vi "Format HF Cell.vi"(0 "PdfP Cell":refnum<k24>, 2 "Header or Footer":T1=enum."Footer", 5 "Header Footer Cluster with references":T2={"Start page"=1, "Type"=enum."Select", "Start with #"=1, "Alignment"=enum."Center", "Vertical Alignement"=enum."MIDDLE", "Page #"={"Text 1"="", "Text 2"="", "Text 3"=""}, "Text"=refnum, "Scaled Img"=refnum, "PdfPCell"=refnum, "PdfPTable"=refnum, "Font Cluster"={"Name"="", "Size"=-1.0, "Color"=0, "Style"={"Bold"=FALSE, "Italic"=FALSE, "Underline"=FALSE, "Strikeout"=FALSE}, "Type"={"Type&direction"=enum."Select", "Embedded"=FALSE, "Encoding"=""}}, "Font "=refnum, "Img (%)"=100.0, "Line"={"Line"=enum."Horizontal line", "Thickness (points)"=0.75, "Colour"=7171459}, "Line spacing"=enum."Select"}, 7 "Padding (points)":sgl, 9 "FixedHeight (points)":sgl, 11 "error in (no error)":errorcluster) -> (4 "PdfP Cell duplicate":refnum<k24>, 15 "error out":errorcluster)   [LabVIEW 2019]
doc: "Version 2.0\nDeveloped by Jean-Marc Simard\nCopyright © 2012, Exaprom Inc.\nAll rights reserved.\nLicense: BSD\n\nWith iTextSharp 4.1.6 (http://itextsharp.sourceforge.net)\nunder Mozilla Public License Version 1.1\n(http://www.mozilla.org/MPL/MPL-1.1.html)"
uses:
  C:/Program Files/National Instruments/LabVIEW 2019/user.lib/Exaprom PDF/DLL/itextsharp.dll
  DLL/itextsharp.dll
  <userlib>/Exaprom PDF/Controls/Header, Footer and Watermark Controls/Header Footer Cluster with references.ctl
  <userlib>/Exaprom PDF/Controls/Header, Footer and Watermark Controls/Header Footer Type.ctl
  <userlib>/Exaprom PDF/Controls/Header, Footer and Watermark Controls/Header footer horiz alignment.ctl
  <userlib>/Exaprom PDF/Controls/Table Controls/Cell Vertical alignment.ctl
  <userlib>/Exaprom PDF/Controls/Header, Footer and Watermark Controls/Page number.ctl
  <userlib>/Exaprom PDF/Controls/Font Controls/Font complete cluster horizontal.ctl
  <userlib>/Exaprom PDF/Controls/Font Controls/Font size.ctl
  <userlib>/Exaprom PDF/Controls/Font Controls/Font color.ctl
  <userlib>/Exaprom PDF/Controls/Font Controls/Type and encoding.ctl
  <userlib>/Exaprom PDF/Controls/Text Controls/Unicode/Type and run direction.ctl
  <userlib>/Exaprom PDF/Controls/Header, Footer and Watermark Controls/Header Footer Line.ctl
  <userlib>/Exaprom PDF/Controls/Text Controls/Line spacing.ctl
  <userlib>/Exaprom PDF/Controls/Header, Footer and Watermark Controls/Header or Footer.ctl
panel:
  # "X"
  # "Y"
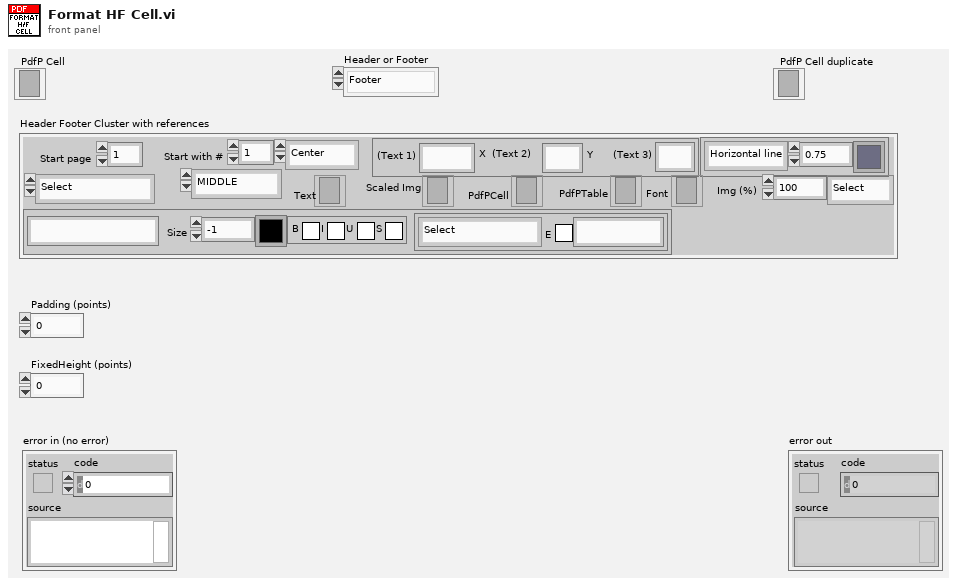
[diagram p1: front panel]
types:
  T1 = typedef "Header or Footer.ctl" = enum16{"Header", "Footer"}
  T2 = typedef "Header Footer Cluster with references.ctl" = cluster{"Start page":i32, "Type":T3, "Start with #":i32, "Alignment":T4, "Vertical Alignement":T5, "Page #":T6, "Text":refnum<k24>, "Scaled Img":refnum<k24>, "PdfPCell":refnum<k24>, "PdfPTable":refnum<k24>, "Font Cluster":T7, "Font ":refnum<k24>, "Img (%)":sgl, "Line":cluster{"Line":T12, "Thickness (points)":sgl, "Colour":T9}, "Line spacing":T13}
  T3 = typedef "Header Footer Type.ctl" = enum16{"Select", "Text", "Text + hyperlink", "Page number", "Image", "Image + hyperlink"}
  T4 = typedef "Header footer horiz alignment.ctl" = enum16{"Left", "Center", "Right"}
  T5 = typedef "Cell Vertical alignment.ctl" = enum16{"TOP", "MIDDLE", "BOTTOM"}
  T6 = typedef "Page number.ctl" = cluster{"Text 1":string, "Text 2":string, "Text 3":string}
  T7 = typedef "Font complete cluster horizontal.ctl" = cluster{"Name":string, "Size":T8, "Color":T9, "Style":cluster{"Bold":bool, "Italic":bool, "Underline":bool, "Strikeout":bool}, "Type":T10}
  T8 = typedef "Font size.ctl" = sgl
  T9 = typedef "Font color.ctl" = u32
  T10 = typedef "Type and encoding.ctl" = cluster{"Type&direction":T11, "Embedded":bool, "Encoding":string}
  T11 = typedef "Type and run direction.ctl" = enum16{"Select", "ASCII", "UTF-16", "UTF-16 (default)", "UTF-16 (LTR)", "UTF-16 (RTL)"}
  T12 = typedef "Header Footer Line.ctl" = enum16{"No line", "Horizontal line"}
  T13 = typedef "Line spacing.ctl" = enum16{"Select", "1.0", "1.5", "2.0"}
  T14 = cluster{"Line":T12, "Thickness (points)":sgl, "Colour":T9}
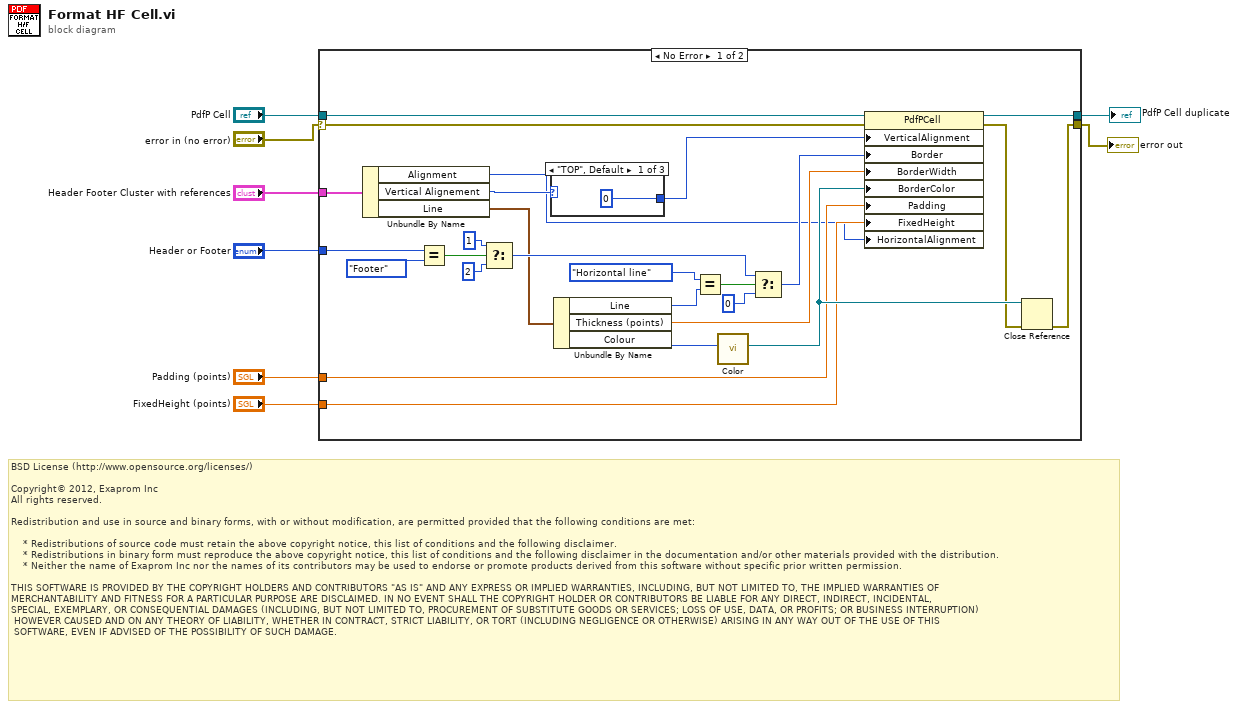
[diagram p0: block diagram]
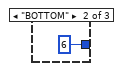
[diagram p2: hidden frame]
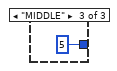
[diagram p3: hidden frame]
diagram:
  # "BSD License (http://www.opensource.org/licenses/)\n\nCopyright© 2012, Exaprom Inc\nAll rights reserved.\n\nRedistribution and use in source and binary forms, with or without modification, are permitted provided that the following conditions are met:\n\n    * Redistributions of source code must retain the above copyright notice, this list of conditions and the following disclaimer.\n    * Redistributions in binary form must reproduce the above copyright notice, this list of conditions and the following disclaimer in the documentation and/or other materials provided with the distribution.\n    * Neither the name of Exaprom Inc nor the names of its contributors may be used to endorse or promote products derived from this software without specific prior written permission.\n\nTHIS SOFTWARE IS PROVIDED BY THE COPYRIGHT HOLDERS AND CONTRIBUTORS \"AS IS\" AND ANY EXPRESS OR IMPLIED WARRANTIES, INCLUDING, BUT NOT LIMITED TO, THE IMPLIED WARRANTIES OF \nMERCHANTABILITY AND FITNESS FOR A PARTICULAR PURPOSE ARE DISCLAIMED. IN NO EVENT SHALL THE COPYRIGHT HOLDER OR CONTRIBUTORS BE LIABLE FOR ANY DIRECT, INDIRECT, INCIDENTAL,\nSPECIAL, EXEMPLARY, OR CONSEQUENTIAL DAMAGES (INCLUDING, BUT NOT LIMITED TO, PROCUREMENT OF SUBSTITUTE GOODS OR SERVICES; LOSS OF USE, DATA, OR PROFITS; OR BUSINESS INTERRUPTION)\n HOWEVER CAUSED AND ON ANY THEORY OF LIABILITY, WHETHER IN CONTRACT, STRICT LIABILITY, OR TORT (INCLUDING NEGLIGENCE OR OTHERWISE) ARISING IN ANY WAY OUT OF THE USE OF THIS\n SOFTWARE, EVEN IF ADVISED OF THE POSSIBILITY OF SUCH DAMAGE."
  n1 = case shown="No Error" "error in (no error)" {
    selector: "error in (no error)" -> [w9 w38]
    tunnel: "PdfP Cell" -> [w19 w39]
    tunnel: [w18 w39] -> w6
    tunnel: [w17 w38] -> w7
    tunnel: "Header Footer Cluster with references" -> [w16 _]
    tunnel: "Padding (points)" -> [w15 _]
    tunnel: "FixedHeight (points)" -> [w14 _]
    tunnel: "Header or Footer" -> [w13 _]
    frame No Error {
      n2 = Unbundle By Name(w16) -> ("Alignment"=w10:T4, "Vertical Alignement"=w24:T5, "Line"=w20:T14)
      n3 = Equal?(x=w13, y=Header_or_Footer."Footer" ("Header or Footer")) -> (x = y?=w30:bool)
      n4 = Select(t=1 ("f"), s=w30, f=2) -> (s? t:f=w33:i32)
      n5 = case shown="\"TOP\", Default" w24 {
        tunnel: [0 6 5] -> w25
        frame "TOP", Default {
        }
        frame "BOTTOM" {
        }
        frame "MIDDLE" {
        }
      }
      n6 = Unbundle By Name(w20) -> ("Line"=w21:T12, "Thickness (points)"=w23:sgl, "Colour"=w28:T9)
      n7 = Equal?(x=Header_Footer_Line."Horizontal line" ("Line"), y=w21) -> (x = y?=w22:bool)
      n8 = call <userlib>:"Color.vi"("Color"=w28) -> ("Color"=w34:refnum<k24>)  [unwired: 1 in, 9 out]
      n9 = Select(t=w33, s=w22, f=0) -> (s? t:f=w11:i32)
      n10 = property class="PdfPCell"(reference=w19, error in=w9, "VerticalAlignment"=w25, "Border"=w11, "BorderWidth"=w23, "BorderColor"=w34, "Padding"=w15, "FixedHeight"=w14, "HorizontalAlignment"=w10) -> (reference out=w18:refnum<k24>, error out=w27:errorcluster)
      n11 = Close Reference(reference=w34, error in (no error)=w27) -> (error out=w17:errorcluster)
    }
    frame Error {
    }
  }
  "error out" <- w7
  "PdfP Cell duplicate" <- w6
